vi "Switch.vi"() -> ()   [LabVIEW 2016]
panel:
  out "Boolean":bool
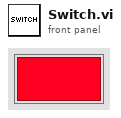
[diagram p1: front panel]
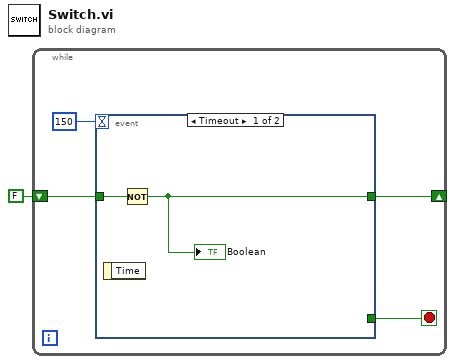
[diagram p0: block diagram]
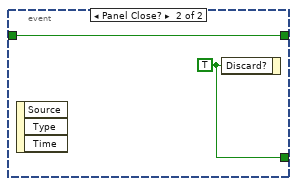
[diagram p2: hidden frame]
diagram:
  n1 = while {
    shift-right: [w4] -> _
    shift-left: FALSE ("Start") -> [w5]
    stop <- w2 stop-if-true
    n2 = event shown="[0] Timeout" {
      selector: _ -> [_ _]
      dyn-events: _ -> [_ _]
      timeout: 150 -> [_ _]
      tunnel: w5 -> [w7 w9]
      tunnel: [w6 w9] -> w4
      tunnel: [_ w8] -> w2
      event Timeout {
        n3 = event-data() -> ()  [unwired: 1 in, 1 out]
        n4 = Not(x=w7) -> (.not. x?=w6:bool)
        "Boolean" <- w6
      }
      event Panel Close? {
        w8 = TRUE ("Discard?")
        n5 = event-data() -> ()  [unwired: 1 in, 3 out]
        n6 = event-data("Discard?"=w8) -> ()  [unwired: 1 in, 1 out]
      }
    }
  }
